vi "4155C Take Sample FPP.vi"(0 "VISA resource name in":refnum<visa-resource-name>, 5 "error in (no error)":errorcluster, 8 "Emergency Stop":refnum<vi>) -> (10 "Time":dbl[](array[numeric]) format="%.2f", 11 "Vp1":dbl[](array[numeric]) format="%.2f", 14 "VISA Resource Name out":refnum<visa-resource-name>, 16 "Ig":dbl[](array[numeric]) format="%.2f", 17 "Id":dbl[](array[numeric]) format="%.2f", 18 "Vp2":dbl[](array[numeric]) format="%.2f", 19 "error out":errorcluster)   [LabVIEW 2016]
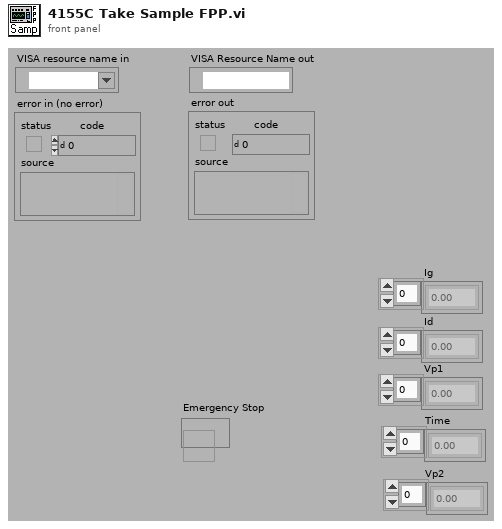
[diagram p1: front panel]
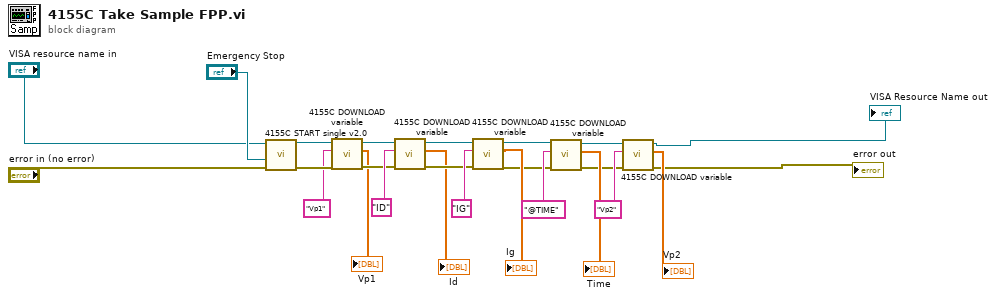
[diagram p0: block diagram]
diagram:
  n1 = call "4155C START single v2.0.vi"("error in (no error)"="error in (no error)", "Emergency Stop"="Emergency Stop", "VISA resource name in"="VISA resource name in") -> ("error out"=w23:errorcluster, "VISA Resource Name out"=w24:refnum<visa-resource-name>)  [unwired: 3 in]
  n2 = call "4155C DOWNLOAD variable.vi"("error in (no error)"=w23, "Variable name"="Vp1", "VISA resource name in"=w24) -> ("error out"=w20:errorcluster, "Output data"=→"Vp1":dbl[], "VISA Resource Name out"=w19:refnum<visa-resource-name>)  [unwired: 2 in]
  n3 = call "4155C DOWNLOAD variable.vi"("error in (no error)"=w20, "Variable name"="ID", "VISA resource name in"=w19) -> ("error out"=w17:errorcluster, "Output data"=→"Id":dbl[], "VISA Resource Name out"=w16:refnum<visa-resource-name>)  [unwired: 2 in]
  n4 = call "4155C DOWNLOAD variable.vi"("error in (no error)"=w17, "Variable name"="IG", "VISA resource name in"=w16) -> ("error out"=w11:errorcluster, "Output data"=→"Ig":dbl[], "VISA Resource Name out"=w12:refnum<visa-resource-name>)  [unwired: 2 in]
  n5 = call "4155C DOWNLOAD variable.vi"("error in (no error)"=w11, "Variable name"="@TIME", "VISA resource name in"=w12) -> ("error out"=w5:errorcluster, "Output data"=→"Time":dbl[], "VISA Resource Name out"=w6:refnum<visa-resource-name>)  [unwired: 2 in]
  n6 = call "4155C DOWNLOAD variable.vi"("error in (no error)"=w5, "Variable name"="Vp2", "VISA resource name in"=w6) -> ("error out"=→"error out":errorcluster, "Output data"=→"Vp2":dbl[], "VISA Resource Name out"=→"VISA Resource Name out":refnum<visa-resource-name>)  [unwired: 2 in]
